vi "FanStop.vi"(11 "VISA resource name":refnum<visa-resource-name>="COM9") -> ()   [LabVIEW 2009]
uses:
  <vilib>/Instr/_visa.llb/VISA Configure Serial Port (Instr).vi
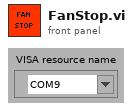
[diagram p1: front panel]
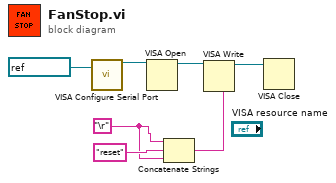
[diagram p0: block diagram]
diagram:
  w1 = "\r"
  n1 = call-poly "VISA Configure Serial Port"("VISA resource name"=refnum<visa-resource-name> "COM9" ("VISA Resource Name")) -> ("VISA resource name out"=w7:refnum<visa-resource-name>)  [unwired: 13 in, 1 out]
  n2 = VISA Open(VISA resource name=w7) -> (VISA resource name=w6:refnum<visa-resource-name>)  [unwired: 4 in, 1 out]
  n3 = Concatenate Strings(w1, "reset", w1) -> (w3:string)
  n4 = VISA Write(VISA resource name=w6, write buffer=w3) -> (VISA resource name out=w2:refnum<visa-resource-name>)  [unwired: 1 in, 2 out]
  n5 = VISA Close(VISA resource name=w2) -> ()  [unwired: 1 in, 1 out]
